vi "(SubVI).vi"(10 "Numeric #2":dbl, 11 "Numeric #1":dbl) -> (3 "Numeric":dbl)   [LabVIEW 2018]
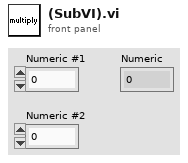
[diagram p1: front panel]
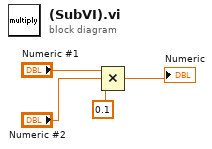
[diagram p0: block diagram]
diagram:
  n1 = Compound Arithmetic op=MULTIPLY("Numeric #1", "Numeric #2", 0.1 ("value")) -> (→"Numeric":dbl)
